vi "Actor Core.vi"(8 "error in":errorcluster, 11 "Nested in":refnum<class "UIActorTop.lvclass">) -> (0 "error out":errorcluster, 3 "Actor out":refnum<class "Actor.lvclass">)   [LabVIEW 2021]
doc: "(<B>Filename</B>: Actor Framework.lvlib:Actor.lvclass:Actor Core.vi)\n\nReceives messages to the actor, reacts to them, and initiates any error handling that may shut the actor down.\n\nDescendant classes may override this VI to append parallel tasks for the actor to complete while it handles messages. Overrides use the Call Parent Method node."
uses:
  <userlib>/John_Lib/AbstractActorTemplate/AbstractActorTemplate/UIActorTop.lvclass
  <vilib>/ActorFramework/Actor/Actor.lvclass
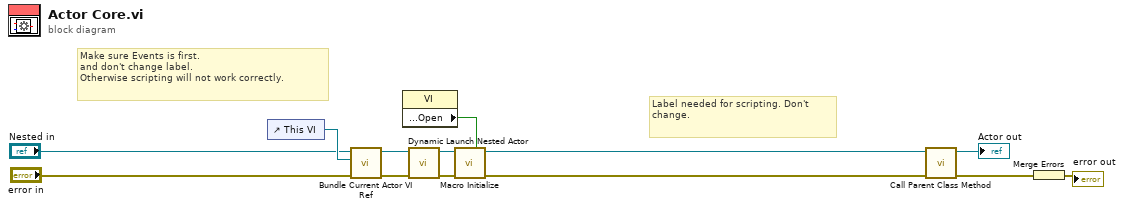
[diagram p0: block diagram]
diagram:
  # "Label needed for scripting. Don't change."
  # "Make sure Events is first.\nand don't change label.\nOtherwise scripting will not work correctly."
  n1 = control-ref of="This VI"() -> (w12:refnum<vi>)
  n2 = call <userlib>:"Bundle Current Actor VI Ref.vi"("error in (no error)"="error in", "This VI"=w12, "UI ActorTop in"="Nested in") -> ("error out"=w8:errorcluster, "UI ActorTop out"=w11:refnum<class "UIActorTop.lvclass">)  [unwired: 6 in, 1 out]
  n3 = property class="VI"() -> ("Front Panel.Open"=w7:bool)  [unwired: 2 in, 2 out]
  n4 = call-dynamic "Dynamic Launch Nested Actor.vi"("error in (no error)"=w8, "UI ActorTop in"=w11) -> ("error out"=w9:errorcluster, "UI ActorTop out"=w10:refnum<class "UIActorTop.lvclass">)  [unwired: 8 in]
  n5 = call-dynamic "Macro Initialize.vi"("Front Panel Window:Open"=w7, "error in (no error)"=w9, "UI ActorTop in"=w10) -> ("error out"=w2:errorcluster, "UI ActorTop out"=w5:refnum<class "UIActorTop.lvclass">)  [unwired: 7 in]
  n6 = call-parent "Call Parent Class Method"("error in"=w2, "Actor in"=w5) -> ("error out"=w4:errorcluster, "Actor out"=→"Actor out":refnum<class "Actor.lvclass">)  [unwired: 8 in]
  n7 = Merge Errors(w4) -> (→"error out":errorcluster)
